vi "sensor cmd memory dump.vi"(6 "dest_buffer_length":i32, 7 "BYTE_ARRAY":string, 9 "num_bytes_to_read":i32, 10 "monitor_memory_address":u32, 11 "device_handle":u32) -> (2 "function return":i32, 3 "device_handle out":u32, 5 "BYTE_ARRAY out":string)   [LabVIEW 2019, in "apdm.lvlib"]
doc: "APDM_EXPORT int apdm_sensor_cmd_memory_dump(apdm_device_handle_t device_handle, const uint32_t monitor_memory_address, const int num_bytes_to_read, char *BYTE_ARRAY, const int dest_buffer_length);"
uses:
  apdm.lvlib
  Lee Lab/CP FES Walking 2018/Code/Working/LabVIEW/apdm.dll
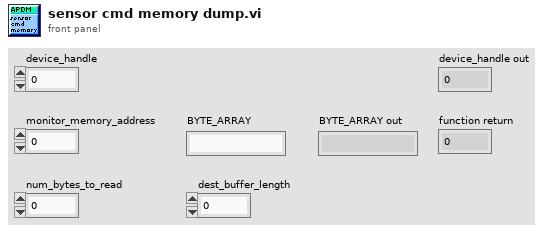
[diagram p1: front panel]
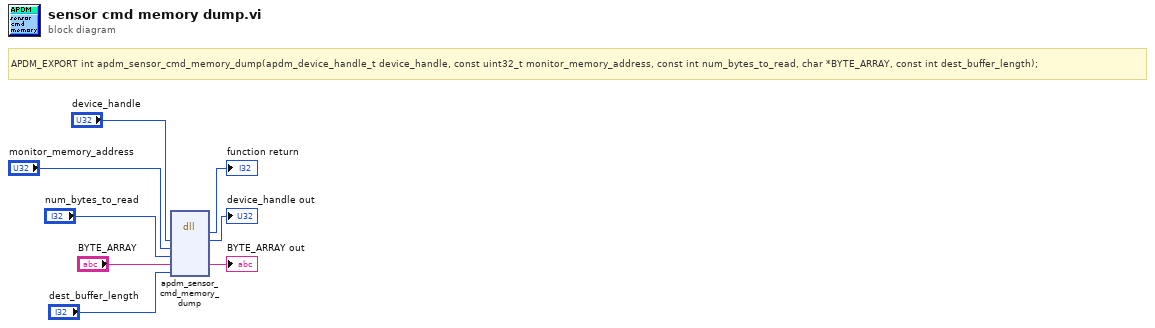
[diagram p0: block diagram]
diagram:
  # "APDM_EXPORT int apdm_sensor_cmd_memory_dump(apdm_device_handle_t device_handle, const uint32_t monitor_memory_address, const int num_bytes_to_read, char *BYTE_ARRAY, const int dest_buffer_length);"
  n1 = dll-call lib="C:/Users/jfalesi/Dropbox/Lee Lab/CP FES Walking 2018/Code/Working/LabVIEW/apdm.*" fn="apdm_sensor_cmd_memory_dump"("device_handle"="device_handle", "monitor_memory_address"="monitor_memory_address", "num_bytes_to_read"="num_bytes_to_read", "BYTE_ARRAY"="BYTE_ARRAY", "dest_buffer_length"="dest_buffer_length") -> (→"function return":i32, "device_handle"=→"device_handle out":u32, "BYTE_ARRAY"=→"BYTE_ARRAY out":string)  [unwired: 6 in, 2 out]
